vi "NI VeriStand - Set Model Execution State.vi"(8 "error in (no error)":errorcluster, 10 "Command":T1 items=["Start", "Pause", "Reset"], 11 "Model in":T2) -> (0 "error out":errorcluster, 3 "Model out":T2)   [LabVIEW 2020, in "NI_VS Model ExecutionAPI.lvlib"]
doc: "Sets the current execution state of the model you specify."
uses:
  <vilib>/NI VeriStand/Execution/Model/NI_VS Model ExecutionAPI.lvlib
  <vilib>/NI VeriStand/Execution/Model/ModelAPI.ctl
  NationalInstruments.VeriStand.ClientAPI
  <vilib>/NI VeriStand/Execution/Model/ModelCommand.ctl
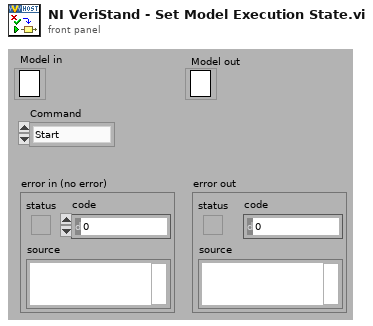
[diagram p1: front panel]
types:
  T1 = typedef "NI_VS Model ExecutionAPI.lvlib/ModelCommand.ctl" = u8
  T2 = typedef "NI_VS Model ExecutionAPI.lvlib/ModelAPI.ctl" = refnum<k24>
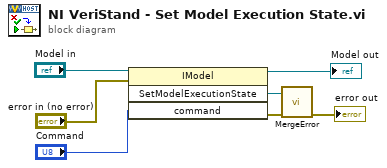
[diagram p0: block diagram]
diagram:
  n1 = invoke class="IModel" method="SetModelExecutionState"(reference="Model in", error in="error in (no error)", "command"="Command") -> (reference out=→"Model out":T2, error out=w5:errorcluster, "SetModelExecutionState"=w4:refnum<k24>)  [unwired: 1 in, 1 out]
  n2 = call <vilib>:"MergeError.vi"("error in (no error)"=w5, "Error"=w4) -> ("error out"=→"error out":errorcluster)  [unwired: 9 out]
